vi "niFPGA Fractional Interval (I32).vi"(7 "direction":u8(ring) items=["falling", "rising"], 9 "y":i32, 10 "y1":i32, 11 "y0":i32) -> (3 "x [U8,0]":u8 format="%.0x")   [LabVIEW 2017]
uses:
  <vilib>/Platform/TimedLoop/XDataNode/timing_clust.ctl
  <vilib>/Platform/TimedLoop/XDataNode/nitl_modes.ctl
  <vilib>/Platform/TimedLoop/XDataNode/wakeup.ctl
  <vilib>/Platform/TimedLoop/XDataNode/XDataNode.xnode
  <vilib>/Platform/TimedLoop/XDataNode/XDNodeRunTimeDep.lvlib
panel:
  # "1-x"
  # "x"
  # "y1"
  # "y"
  # "y0"
  # "0"
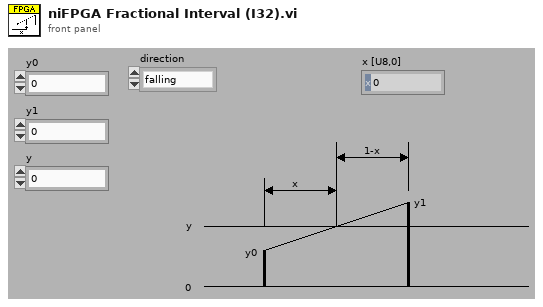
[diagram p1: front panel]
types:
  T1 = typedef "XDNodeRunTimeDep.lvlib/timing_clust.ctl" = cluster{"Expected End [f-1]":u64, "Actual End [f-1]":u64, "Finished Late? [f-1]":bool, "Expected End [i-1]":u64, "Actual End [i-1]":u64, "Finished Late? [i-1]":bool, "Expected Start [i]":u64, "Actual Start [i]":u64, "Expected Start [f]":u64, "Actual Start [f]":u64, "Source Name":string, "Structure Name":string, "Period":i64, "Deadline":i64, "Offset":i64, "Start":i64, "Priority":i32, "Timeout":i32, "Mode":T2, "Wakeup Reason":T3, "Error":errorcluster, "Source Type":string, "Secondary Source Type":string, "Global End Time":u64, "Global Start Time":u64, "Frame Duration":u64, "Iteration Duration":u64, "Assigned CPU":i32, "I/O Scan Engine Mode":u32}
  T2 = typedef "XDNodeRunTimeDep.lvlib/nitl_modes.ctl" = enum32{"No Change", "Process missed periods, maintain original phase", "Discard missed periods, maintain original phase", "Process missed periods, ignore original phase", "Discard missed periods, ignore original phase"}
  T3 = typedef "XDNodeRunTimeDep.lvlib/wakeup.ctl" = enum32{"Normal", "Aborted", "Asynchronous wakeup", "Timing source error", "Timed loop error", "Timeout"}
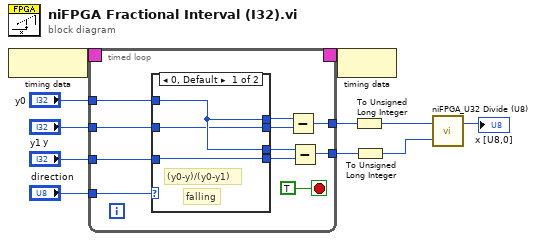
[diagram p0: block diagram]
diagram:
  n1 = node-c288() -> (w11:T1)
  n2 = timed-loop {
    timing: w11 -> [_]
    timing-out: [_] -> w10
    tunnel: "y1" -> [w18]
    tunnel: "y" -> [w21]
    tunnel: "y0" -> [w20]
    tunnel: "direction" -> [w19]
    tunnel: [w13] -> w5
    tunnel: [w12] -> w4
    stop <- TRUE stop-if-true
    n3 = case shown="0, Default" w19 {
      tunnel: [w24 w28] -> w17
      tunnel: w21 -> [w23 w27]
      tunnel: w20 -> [w24 w26]
      tunnel: w18 -> [w25 w28]
      tunnel: [w25 w26] -> w16
      tunnel: [w24 w27] -> w15
      tunnel: [w23 w26] -> w14
      frame 0, Default {
        # "(y0-y)/(y0-y1)"
        # "falling"
      }
      frame 1 {
        # "(y-y0)/(y1-y0)"
        # "rising"
      }
    }
    n4 = Subtract(x=w15, y=w14) -> (x-y=w12:i32)
    n5 = Subtract(x=w17, y=w16) -> (x-y=w13:i32)
  }
  n6 = node-c288(w10) -> ()
  n7 = To Unsigned Long Integer(number=w4) -> (unsigned 32bit integer=w2:u32)
  n8 = To Unsigned Long Integer(number=w5) -> (unsigned 32bit integer=w3:u32)
  n9 = call <vilib>:"niFPGA_U32 Divide (U8).vi"("D [U32.n]"=w3, "N [U32.n]"=w2) -> ("N/D [U8.0]"=→"x [U8,0]":u8)  [unwired: 1 out]
